vi "Unpack welcome byte.vi"(8 "error in":errorcluster, 11 "Byte":u8[](array[numeric]) format="%x") -> (0 "error (out)":errorcluster, 2 "Serialisation":T1=1 items=["JSON"=1, "MessagePack"=2], 3 "Length (octets)":u8 format="%b")   [LabVIEW 2020, in "wamplv.lvlib" / "RawSocket Handler.lvclass"]
uses:
  RawSocket Handler.lvclass
  <vilib>/Utility/error.llb/Error Cluster From Error Code.vi
  <vilib>/ErrorRing/Error Ring.xnode
  Serilisation Types.ctl
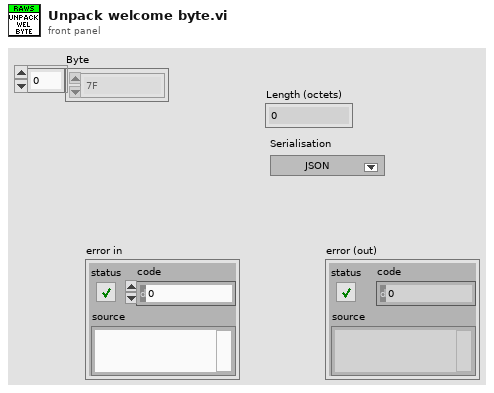
[diagram p1: front panel]
types:
  T1 = typedef "wamplv.lvlib/RawSocket Handler.lvclass/Serilisation Types.ctl" = u8
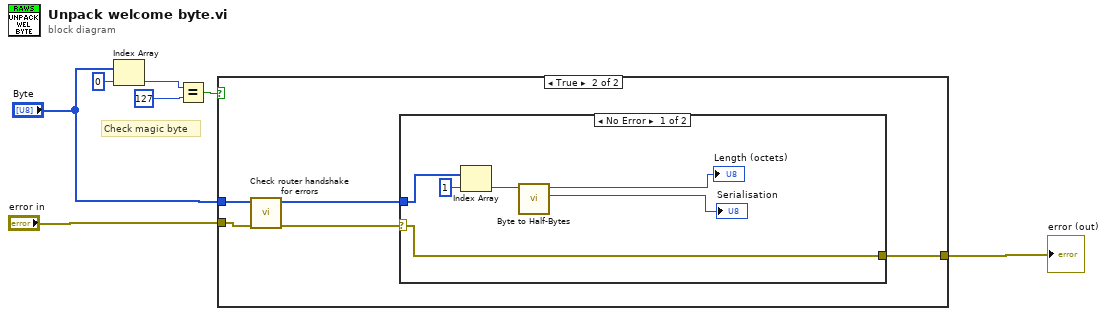
[diagram p0: block diagram]
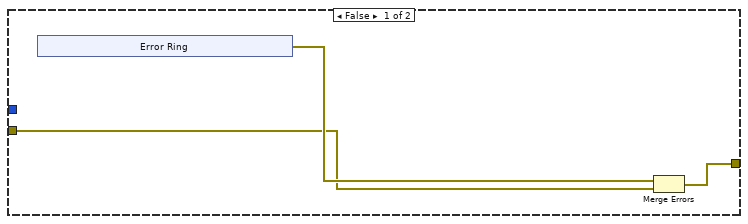
[diagram p2: hidden frame]
diagram:
  # "Check magic byte"
  n1 = Index Array(array="Byte", index=0) -> (element=w5:u8)
  n2 = Equal?(x=w5, y=u8 127) -> (x = y?=w4:bool)
  n3 = case shown="True" w4 {
    tunnel: "Byte" -> [_ w19]
    tunnel: [w9 w15] -> w1
    tunnel: "error in" -> [w8 w18]
    frame False {
      n4 = xnode "Error Ring"() -> ("error out"=w10:errorcluster)
      n5 = Merge Errors(w10, w8) -> (w9:errorcluster)
    }
    frame True {
      n6 = call "Check router handshake for errors.vi"("error in"=w18, "Bytes (in)"=w19) -> ("error out"=w17:errorcluster, "Byte (out)"=w16:u8[])  [unwired: 8 in]
      n7 = case shown="No Error" w17 {
        selector: w17 -> [w22 w26]
        tunnel: w16 -> [w25 _]
        tunnel: [w22 w26] -> w15
        frame No Error {
          n8 = Index Array(array=w25, index=1) -> (element=w23:u8)
          n9 = call "Byte to Half-Bytes.vi"("Byte In"=w23) -> ("Lower Half-byte"=→"Serialisation":u8, "Upper Half-Byte"=→"Length (octets)":u8)  [unwired: 7 in]
        }
        frame Error {
        }
      }
    }
  }
  "error (out)" <- w1
